vi "FA_ConvertFromConfigData.vi"(8 "Error In":errorcluster, 11 "Config":T1) -> (0 "Error Out":errorcluster, 3 "XML String":string)   [LabVIEW 2014, in "FA_NativeTypes.lvlib"]
doc: "Converts a LabVIEW cluster describing a configuration into XML text"
uses:
  FA_NativeTypes.lvlib
  FA_LocalStore API/source/VI Source/FA_LSSpecialTypes.ctl
  FA_LocalStore API/source/VI Source/FA_LocalStore.lvlib
  FA_Config.ctl
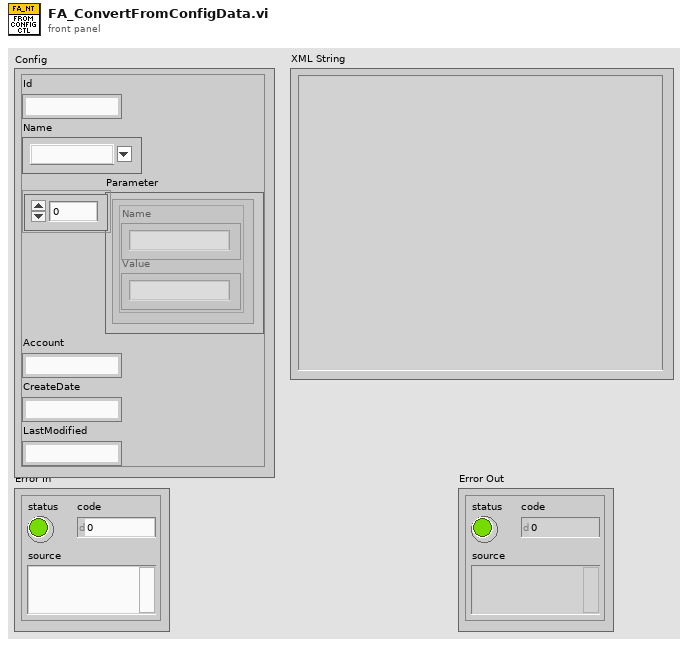
[diagram p1: front panel]
types:
  T1 = typedef "FA_NativeTypes.lvlib/FA_Config.ctl" = cluster{"Id":string, "Name":T2, "Parameter":cluster{"Name":string, "Value":string}[], "Account":string, "CreateDate":string, "LastModified":string}
  T2 = typedef "FA_LocalStore.lvlib/FA_LSSpecialTypes.ctl" = string
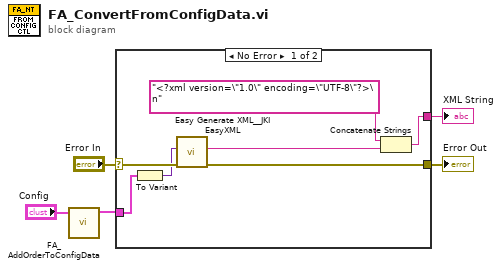
[diagram p0: block diagram]
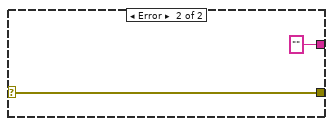
[diagram p2: hidden frame]
diagram:
  n1 = call "FA_AddOrderToConfigData.vi"("Config in"="Config") -> ("Config"=w1:T1)  [unwired: 10 in]
  n2 = case shown="No Error" "Error In" {
    selector: "Error In" -> [w12 w14]
    tunnel: [w10 w14] -> w5
    tunnel: [w6 "" ("XML String")] -> w3
    tunnel: w1 -> [w9 _]
    frame No Error {
      n3 = To Variant(anything=w9) -> (Variant=w11:variant)
      n4 = call <vilib>:"Easy Generate XML__JKI EasyXML.vi"("error in (no error)"=w12, "LabVIEW Data"=w11) -> ("error out"=w10:errorcluster, "XML String"=w7:string)  [unwired: 8 in]
      n5 = Concatenate Strings("<?xml version=\"1.0\" encoding=\"UTF-8\"?>\n" ("string"), w7) -> (w6:string)
    }
    frame Error {
    }
  }
  "Error Out" <- w5
  "XML String" <- w3
